vi "Age.vi"(11 "Atom In":refnum<class "Atom.lvclass">) -> (2 "Current Age":i32, 3 "Atom Out":refnum<class "Atom.lvclass">)   [LabVIEW 2020, in "Atom.lvclass"]
uses:
  Atom.lvclass
  Atom.lvclass/Atom.ctl
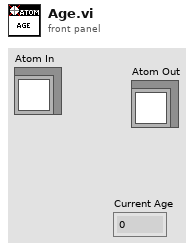
[diagram p1: front panel]
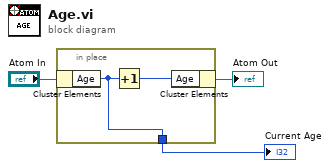
[diagram p0: block diagram]
diagram:
  n1 = in-place {
    in-place-border: [w4] -> w1
    n2 = in-place-cluster #1("Atom In") -> ("Age"=w4:i32)
    n3 = Increment(x=w4) -> (x+1=w5:i32)
    n4 = in-place-cluster #1("Age"=w5) -> (→"Atom Out":refnum<class "Atom.lvclass">)
  }
  "Current Age" <- w1
